vi "Set Tuner IF Gain.vi"(8 "error in (no error)":errorcluster, 9 "Gain (dB)":dbl, 10 "Stage":i32, 11 "DeviceRefnum":u64) -> (0 "error out":errorcluster, 2 "function return":i32, 3 "DeviceRefnum Out":u64)   [LabVIEW 2014]
doc: "Set the intermediate frequency gain for the device."
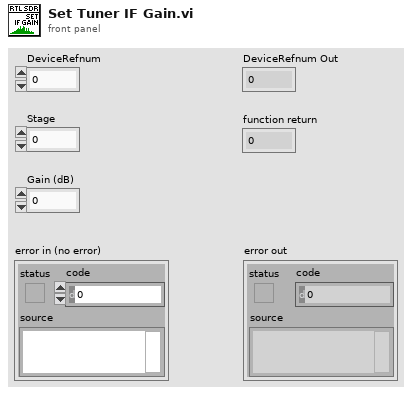
[diagram p1: front panel]
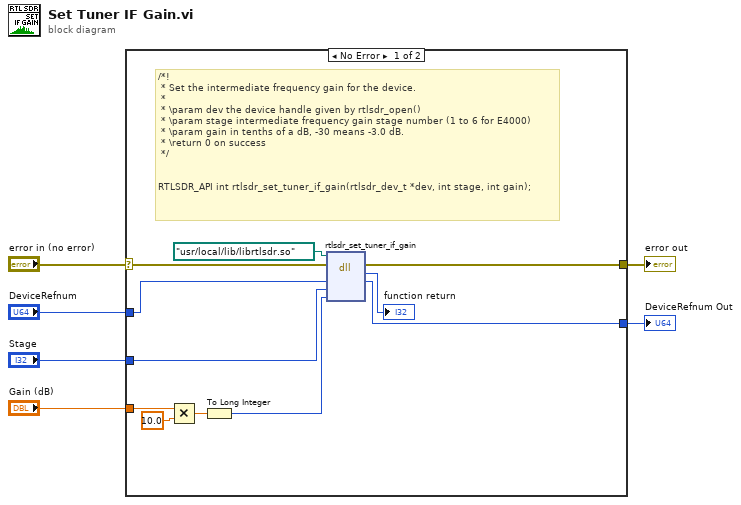
[diagram p0: block diagram]
diagram:
  n1 = case shown="No Error" "error in (no error)" {
    selector: "error in (no error)" -> [w9 w19]
    tunnel: "Stage" -> [w16 _]
    tunnel: "DeviceRefnum" -> [w15 w18]
    tunnel: [w14 w18] -> w4
    tunnel: "Gain (dB)" -> [w13 _]
    tunnel: [w7 w19] -> w1
    frame No Error {
      # "/*!\n * Set the intermediate frequency gain for the device.\n *\n * \\param dev the device handle given by rtlsdr_open()\n * \\param stage intermediate frequency gain stage number (1 to 6 for E4000)\n * \\param gain in tenths of a dB, -30 means -3.0 dB.\n * \\return 0 on success\n */\n\n\nRTLSDR_API int rtlsdr_set_tuner_if_gain(rtlsdr_dev_t *dev, int stage, int gain);"
      n2 = Multiply(x=w13, y=10.0) -> (x*y=w11:dbl)
      n3 = To Long Integer(number=w11) -> (32bit integer=w10:i32)
      n4 = dll-call lib="C:/Program Files (x86)/National Instruments/LabVIEW 2016/user.lib/rtlsdr/rtlsdr.*" fn="rtlsdr_set_tuner_if_gain"(path in=path "/usr/local/lib/librtlsdr.so", error in=w9, "DeviceRefnum"=w15, "Stage"=w16, "Gain"=w10) -> (error out=w7:errorcluster, "return type"=→"function return":i32, "DeviceRefnum"=w14:u64)  [unwired: 3 in, 1 out]
    }
    frame Error {
    }
  }
  "DeviceRefnum Out" <- w4
  "error out" <- w1
